vi "set_objectArray.vi"(0 "HGF_ThreadTask":refnum<class "HGF_ThreadTask.lvclass">, 2 "objectArray":refnum<class "HGF_Visitable.lvclass">[](array[class]), 3 "errorArray":errorcluster[](array[cluster]), 5 "error in (no error)":errorcluster) -> (14 "dup HGF_ThreadTask":refnum<class "HGF_ThreadTask.lvclass">, 19 "error out":errorcluster)   [LabVIEW 2014, in "HGF_BaseClasses.lvlib" / "HGF_ThreadTask.lvclass"]
doc: "Write object array."
uses:
  HGF_ThreadTask.lvclass
  HGF_Visitable/HGF_Visitable.lvclass
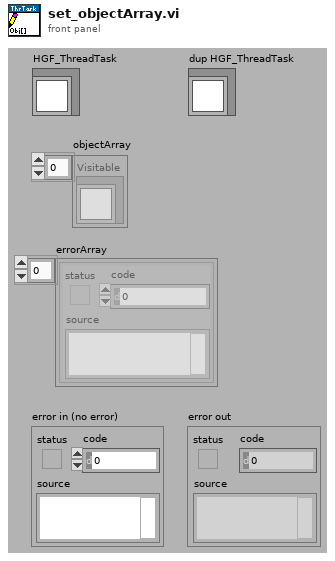
[diagram p1: front panel]
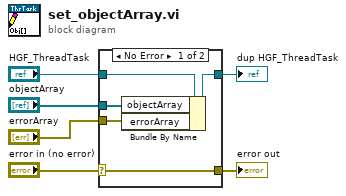
[diagram p0: block diagram]
diagram:
  n1 = case shown="No Error" "error in (no error)" {
    selector: "error in (no error)" -> [w11 w12]
    tunnel: [w11 w12] -> w5
    tunnel: [w9 w13] -> w3
    tunnel: "HGF_ThreadTask" -> [w10 w13]
    tunnel: "objectArray" -> [w8 _]
    tunnel: "errorArray" -> [w7 _]
    frame No Error {
      n2 = Bundle By Name(cluster=w10, "objectArray"=w8, "errorArray"=w7) -> (w9:refnum<class "HGF_ThreadTask.lvclass">)
    }
    frame Error {
    }
  }
  "error out" <- w5
  "dup HGF_ThreadTask" <- w3
